vi "testRawXmlNestedCluster.vi"(8 "error in (no error)":errorcluster, 11 "TestCase in":refnum<class "EasyXMLTest.lvclass">) -> (0 "error out":errorcluster, 3 "TestCase out":refnum<class "EasyXMLTest.lvclass">)   [LabVIEW 2011, in "EasyXMLTest.lvclass"]
doc: "Verify that error in is not overwritten"
uses:
  EasyXMLTest.lvclass
panel:
  out "data":T1
  out "Produced Data":variant
  out "Input Data":variant
  out "XML String":string
  out "Generated XML String":string
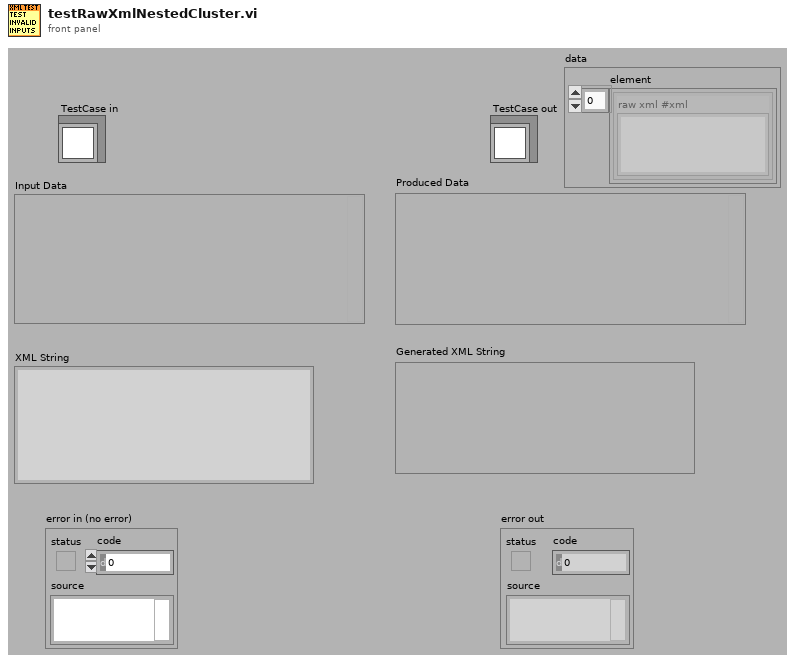
[diagram p1: front panel]
types:
  T1 = cluster{"element":cluster{"raw xml #xml":string}[]}
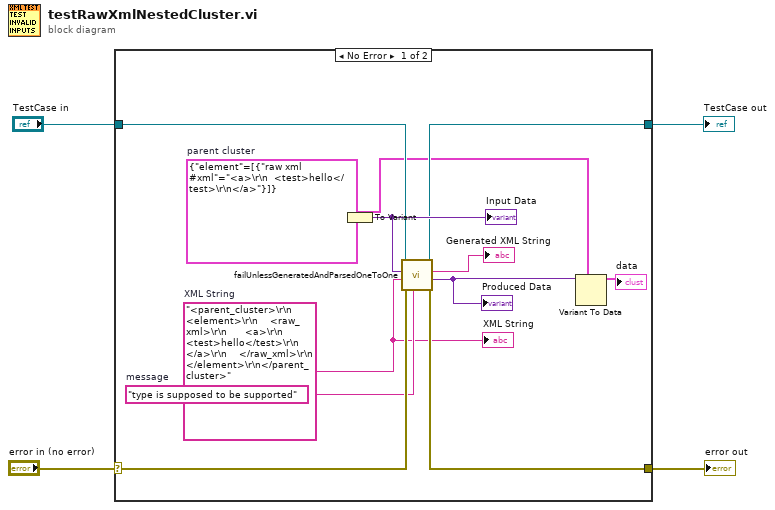
[diagram p0: block diagram]
diagram:
  n1 = case shown="No Error" "error in (no error)" {
    selector: "error in (no error)" -> [w14 w17]
    tunnel: [w10 w17] -> w2
    tunnel: [w9 w16] -> w1
    tunnel: "TestCase in" -> [w15 w16]
    frame No Error {
      w6 = T1 {"element"=[{"raw xml #xml"="<a>\r\n  <test>hello</test>\r\n</a>"}]}  # parent cluster
      w8 = "<parent_cluster>\r\n  <element>\r\n    <raw_xml>\r\n      <a>\r\n        <test>hello</test>\r\n      </a>\r\n    </raw_xml>\r\n  </element>\r\n</parent_cluster>"  # XML String
      w13 = "type is supposed to be supported"  # message
      n2 = To Variant(anything=w6) -> (Variant=w12:variant)
      "Input Data" <- w12
      n3 = call "failUnlessGeneratedAndParsedOneToOne.vi"("message (\"\")"=w13, "error in"=w14, "XML String"=w8, "Data"=w12, "EasyXMLTest in"=w15) -> ("error out"=w10:errorcluster, "Produced Data"=w7:variant, "Generated XML String"=→"Generated XML String":string, "EasyXMLTest out"=w9:refnum<class "EasyXMLTest.lvclass">)  [unwired: 3 in]
      "Produced Data" <- w7
      n4 = Variant To Data(type=w6, Variant=w7) -> (data=→"data":T1)  [unwired: 1 in, 1 out]
      "XML String" <- w8
    }
    frame Error {
    }
  }
  "error out" <- w2
  "TestCase out" <- w1
